vi "Generate Error.vi"(8 "Error In":errorcluster, 11 "Error Type":T1) -> (0 "Error Out":errorcluster)   [LabVIEW 2011, in "LVH-Adept.lvlib" / "DMGR.lvlib"]
uses:
  DMGR.lvlib
  Type Defs/Error.ctl
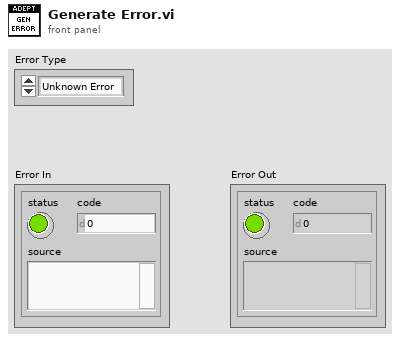
[diagram p1: front panel]
types:
  T1 = typedef "LVH-Adept.lvlib/DMGR.lvlib/Error.ctl" = enum16{"Unknown Error", "Device Enumeration", "Device Handle", "Device Info", "Device Open"}
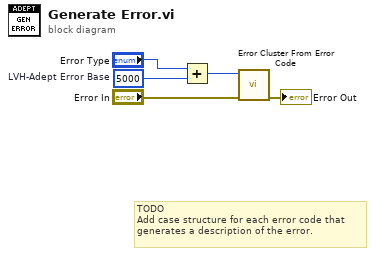
[diagram p0: block diagram]
diagram:
  w4 = 5000  # LVH-Adept Error Base
  # "TODO\nAdd case structure for each error code that \ngenerates a description of the error."
  n1 = Add(x="Error Type", y=w4) -> (x+y=w2:i32)
  n2 = call <vilib>:"Error Cluster From Error Code.vi"("error in (no error)"="Error In", "error code (0)"=w2) -> ("error out"=→"Error Out":errorcluster)  [unwired: 7 in]
